vi "Pipeline Boolean Signal.vi"(7 "reset":bool, 10 "delay":fxp<+,5,5>, 11 "input signal":bool) -> (3 "output signal":bool)   [LabVIEW 2018]
doc: "Provide controlled delay for boolean signal."
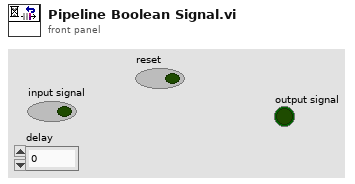
[diagram p1: front panel]
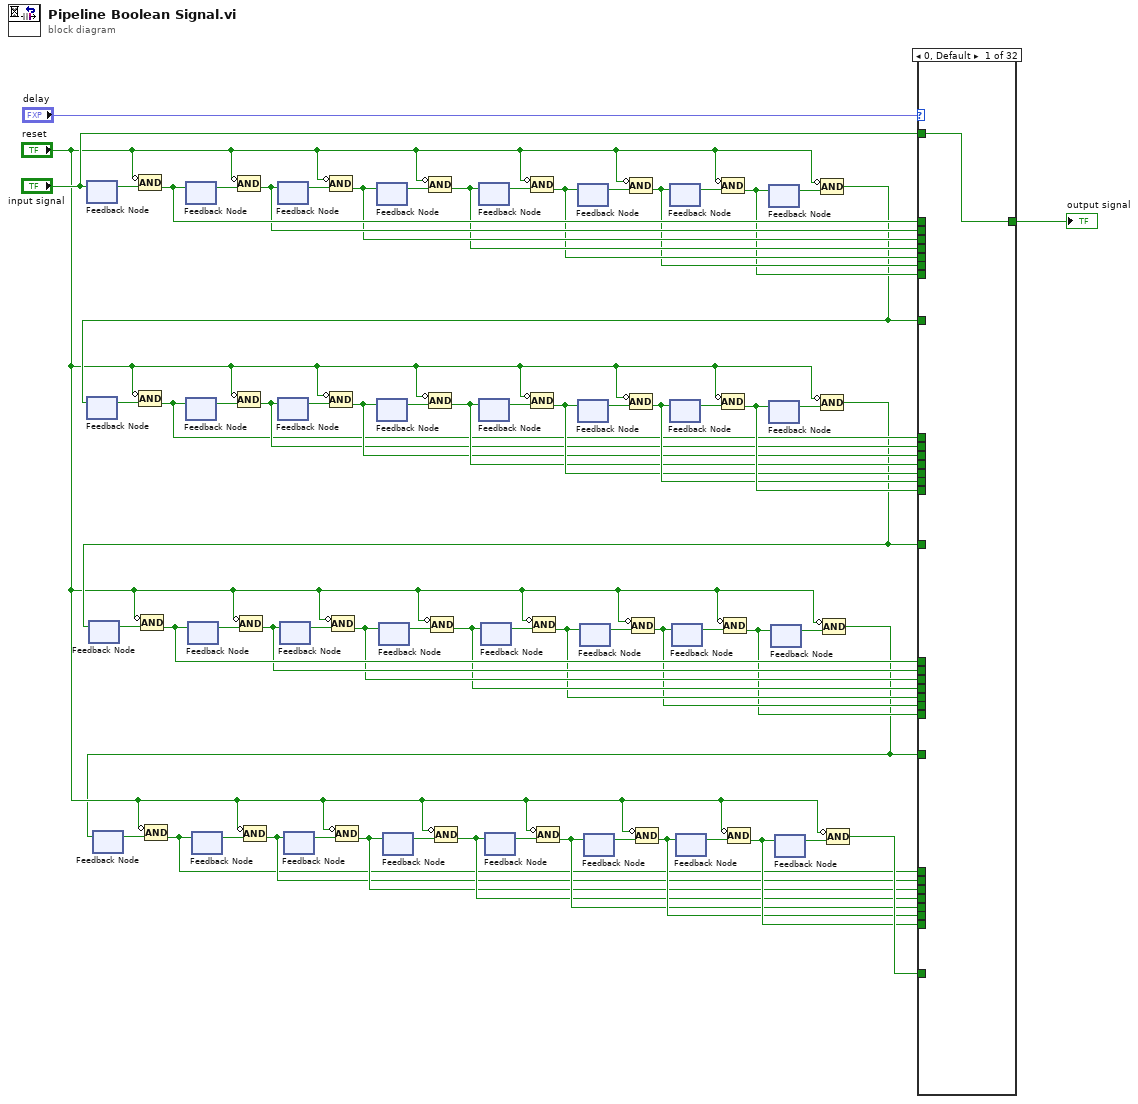
[diagram p0: block diagram]
diagram:
  n1 = feedback-in #1("input signal") -> ()
  n2 = feedback #1() -> (w65:bool)  [unwired: 1 in]
  n3 = feedback #2() -> (w41:bool)  [unwired: 1 in]
  n4 = feedback #3() -> (w31:bool)  [unwired: 1 in]
  n5 = feedback #4() -> (w6:bool)  [unwired: 1 in]
  n6 = Compound Arithmetic op=AND(invert "reset", w65) -> (w64:bool)
  n7 = Compound Arithmetic op=AND(invert "reset", w41) -> (w42:bool)
  n8 = Compound Arithmetic op=AND(invert "reset", w31) -> (w30:bool)
  n9 = Compound Arithmetic op=AND(invert "reset", w6) -> (w7:bool)
  n10 = feedback #5() -> (w68:bool)  [unwired: 1 in]
  n11 = feedback-in #5(w64) -> ()
  n12 = feedback #6() -> (w38:bool)  [unwired: 1 in]
  n13 = feedback-in #6(w42) -> ()
  n14 = feedback #7() -> (w34:bool)  [unwired: 1 in]
  n15 = feedback-in #7(w30) -> ()
  n16 = feedback #8() -> (w3:bool)  [unwired: 1 in]
  n17 = feedback-in #8(w7) -> ()
  n18 = Compound Arithmetic op=AND(invert "reset", w68) -> (w63:bool)
  n19 = Compound Arithmetic op=AND(invert "reset", w38) -> (w43:bool)
  n20 = Compound Arithmetic op=AND(invert "reset", w34) -> (w29:bool)
  n21 = Compound Arithmetic op=AND(invert "reset", w3) -> (w8:bool)
  n22 = feedback #9() -> (w67:bool)  [unwired: 1 in]
  n23 = feedback-in #9(w63) -> ()
  n24 = feedback #10() -> (w39:bool)  [unwired: 1 in]
  n25 = feedback-in #10(w43) -> ()
  n26 = feedback #11() -> (w33:bool)  [unwired: 1 in]
  n27 = feedback-in #11(w29) -> ()
  n28 = feedback #12() -> (w4:bool)  [unwired: 1 in]
  n29 = feedback-in #12(w8) -> ()
  n30 = Compound Arithmetic op=AND(invert "reset", w67) -> (w62:bool)
  n31 = Compound Arithmetic op=AND(invert "reset", w39) -> (w44:bool)
  n32 = Compound Arithmetic op=AND(invert "reset", w33) -> (w28:bool)
  n33 = Compound Arithmetic op=AND(invert "reset", w4) -> (w9:bool)
  n34 = feedback #13() -> (w66:bool)  [unwired: 1 in]
  n35 = feedback-in #13(w62) -> ()
  n36 = feedback #14() -> (w40:bool)  [unwired: 1 in]
  n37 = feedback-in #14(w44) -> ()
  n38 = feedback #15() -> (w32:bool)  [unwired: 1 in]
  n39 = feedback-in #15(w28) -> ()
  n40 = feedback #16() -> (w5:bool)  [unwired: 1 in]
  n41 = feedback-in #16(w9) -> ()
  n42 = Compound Arithmetic op=AND(invert "reset", w66) -> (w57:bool)
  n43 = Compound Arithmetic op=AND(invert "reset", w40) -> (w49:bool)
  n44 = Compound Arithmetic op=AND(invert "reset", w32) -> (w23:bool)
  n45 = Compound Arithmetic op=AND(invert "reset", w5) -> (w14:bool)
  n46 = feedback #17() -> (w61:bool)  [unwired: 1 in]
  n47 = feedback-in #17(w57) -> ()
  n48 = feedback #18() -> (w45:bool)  [unwired: 1 in]
  n49 = feedback-in #18(w49) -> ()
  n50 = feedback #19() -> (w27:bool)  [unwired: 1 in]
  n51 = feedback-in #19(w23) -> ()
  n52 = feedback #20() -> (w10:bool)  [unwired: 1 in]
  n53 = feedback-in #20(w14) -> ()
  n54 = Compound Arithmetic op=AND(invert "reset", w61) -> (w56:bool)
  n55 = Compound Arithmetic op=AND(invert "reset", w45) -> (w50:bool)
  n56 = Compound Arithmetic op=AND(invert "reset", w27) -> (w22:bool)
  n57 = Compound Arithmetic op=AND(invert "reset", w10) -> (w15:bool)
  n58 = feedback #21() -> (w58:bool)  [unwired: 1 in]
  n59 = feedback-in #21(w56) -> ()
  n60 = feedback #22() -> (w48:bool)  [unwired: 1 in]
  n61 = feedback-in #22(w50) -> ()
  n62 = feedback #23() -> (w24:bool)  [unwired: 1 in]
  n63 = feedback-in #23(w22) -> ()
  n64 = feedback #24() -> (w13:bool)  [unwired: 1 in]
  n65 = feedback-in #24(w15) -> ()
  n66 = Compound Arithmetic op=AND(invert "reset", w58) -> (w55:bool)
  n67 = Compound Arithmetic op=AND(invert "reset", w48) -> (w51:bool)
  n68 = Compound Arithmetic op=AND(invert "reset", w24) -> (w21:bool)
  n69 = Compound Arithmetic op=AND(invert "reset", w13) -> (w16:bool)
  n70 = feedback #25() -> (w59:bool)  [unwired: 1 in]
  n71 = feedback-in #25(w55) -> ()
  n72 = feedback #26() -> (w47:bool)  [unwired: 1 in]
  n73 = feedback-in #26(w51) -> ()
  n74 = feedback #27() -> (w25:bool)  [unwired: 1 in]
  n75 = feedback-in #27(w21) -> ()
  n76 = feedback #28() -> (w12:bool)  [unwired: 1 in]
  n77 = feedback-in #28(w16) -> ()
  n78 = Compound Arithmetic op=AND(invert "reset", w59) -> (w54:bool)
  n79 = Compound Arithmetic op=AND(invert "reset", w47) -> (w52:bool)
  n80 = Compound Arithmetic op=AND(invert "reset", w25) -> (w20:bool)
  n81 = Compound Arithmetic op=AND(invert "reset", w12) -> (w17:bool)
  n82 = feedback #29() -> (w60:bool)  [unwired: 1 in]
  n83 = feedback-in #29(w54) -> ()
  n84 = feedback #30() -> (w46:bool)  [unwired: 1 in]
  n85 = feedback-in #30(w52) -> ()
  n86 = feedback #31() -> (w26:bool)  [unwired: 1 in]
  n87 = feedback-in #31(w20) -> ()
  n88 = feedback #32() -> (w11:bool)  [unwired: 1 in]
  n89 = feedback-in #32(w17) -> ()
  n90 = Compound Arithmetic op=AND(invert "reset", w60) -> (w37:bool)
  n91 = feedback-in #2(w37) -> ()
  n92 = Compound Arithmetic op=AND(invert "reset", w46) -> (w19:bool)
  n93 = feedback-in #3(w19) -> ()
  n94 = Compound Arithmetic op=AND(invert "reset", w26) -> (w1:bool)
  n95 = feedback-in #4(w1) -> ()
  n96 = Compound Arithmetic op=AND(invert "reset", w11) -> (w18:bool)
  n97 = case shown="0, Default" "delay" {
    tunnel: w64 -> [_ w70 _ _ _ _ _ _ _ _ _ _ _ _ _ _ _ _ _ _ _ _ _ _ _ _ _ _ _ _ _ _]
    tunnel: w63 -> [_ _ w71 _ _ _ _ _ _ _ _ _ _ _ _ _ _ _ _ _ _ _ _ _ _ _ _ _ _ _ _ _]
    tunnel: w62 -> [_ _ _ w72 _ _ _ _ _ _ _ _ _ _ _ _ _ _ _ _ _ _ _ _ _ _ _ _ _ _ _ _]
    tunnel: w57 -> [_ _ _ _ w73 _ _ _ _ _ _ _ _ _ _ _ _ _ _ _ _ _ _ _ _ _ _ _ _ _ _ _]
    tunnel: w56 -> [_ _ _ _ _ w74 _ _ _ _ _ _ _ _ _ _ _ _ _ _ _ _ _ _ _ _ _ _ _ _ _ _]
    tunnel: w55 -> [_ _ _ _ _ _ w75 _ _ _ _ _ _ _ _ _ _ _ _ _ _ _ _ _ _ _ _ _ _ _ _ _]
    tunnel: w54 -> [_ _ _ _ _ _ _ w76 _ _ _ _ _ _ _ _ _ _ _ _ _ _ _ _ _ _ _ _ _ _ _ _]
    tunnel: [w69 w70 w71 w72 w73 w74 w75 w76 w77 w78 w79 w80 w81 w82 w83 w84 w85 w86 w87 w88 w89 w90 w91 w92 w93 w94 w95 w96 w97 w98 w99 w100] -> w53
    tunnel: w37 -> [_ _ _ _ _ _ _ _ w77 _ _ _ _ _ _ _ _ _ _ _ _ _ _ _ _ _ _ _ _ _ _ _]
    tunnel: w42 -> [_ _ _ _ _ _ _ _ _ w78 _ _ _ _ _ _ _ _ _ _ _ _ _ _ _ _ _ _ _ _ _ _]
    tunnel: w43 -> [_ _ _ _ _ _ _ _ _ _ w79 _ _ _ _ _ _ _ _ _ _ _ _ _ _ _ _ _ _ _ _ _]
    tunnel: w44 -> [_ _ _ _ _ _ _ _ _ _ _ w80 _ _ _ _ _ _ _ _ _ _ _ _ _ _ _ _ _ _ _ _]
    tunnel: w49 -> [_ _ _ _ _ _ _ _ _ _ _ _ w81 _ _ _ _ _ _ _ _ _ _ _ _ _ _ _ _ _ _ _]
    tunnel: w50 -> [_ _ _ _ _ _ _ _ _ _ _ _ _ w82 _ _ _ _ _ _ _ _ _ _ _ _ _ _ _ _ _ _]
    tunnel: w51 -> [_ _ _ _ _ _ _ _ _ _ _ _ _ _ w83 _ _ _ _ _ _ _ _ _ _ _ _ _ _ _ _ _]
    tunnel: w52 -> [_ _ _ _ _ _ _ _ _ _ _ _ _ _ _ w84 _ _ _ _ _ _ _ _ _ _ _ _ _ _ _ _]
    tunnel: "input signal" -> [w69 _ _ _ _ _ _ _ _ _ _ _ _ _ _ _ _ _ _ _ _ _ _ _ _ _ _ _ _ _ _ _]
    tunnel: w19 -> [_ _ _ _ _ _ _ _ _ _ _ _ _ _ _ _ w85 _ _ _ _ _ _ _ _ _ _ _ _ _ _ _]
    tunnel: w30 -> [_ _ _ _ _ _ _ _ _ _ _ _ _ _ _ _ _ w86 _ _ _ _ _ _ _ _ _ _ _ _ _ _]
    tunnel: w29 -> [_ _ _ _ _ _ _ _ _ _ _ _ _ _ _ _ _ _ w87 _ _ _ _ _ _ _ _ _ _ _ _ _]
    tunnel: w28 -> [_ _ _ _ _ _ _ _ _ _ _ _ _ _ _ _ _ _ _ w88 _ _ _ _ _ _ _ _ _ _ _ _]
    tunnel: w23 -> [_ _ _ _ _ _ _ _ _ _ _ _ _ _ _ _ _ _ _ _ w89 _ _ _ _ _ _ _ _ _ _ _]
    tunnel: w22 -> [_ _ _ _ _ _ _ _ _ _ _ _ _ _ _ _ _ _ _ _ _ w90 _ _ _ _ _ _ _ _ _ _]
    tunnel: w21 -> [_ _ _ _ _ _ _ _ _ _ _ _ _ _ _ _ _ _ _ _ _ _ w91 _ _ _ _ _ _ _ _ _]
    tunnel: w20 -> [_ _ _ _ _ _ _ _ _ _ _ _ _ _ _ _ _ _ _ _ _ _ _ w92 _ _ _ _ _ _ _ _]
    tunnel: w1 -> [_ _ _ _ _ _ _ _ _ _ _ _ _ _ _ _ _ _ _ _ _ _ _ _ w93 _ _ _ _ _ _ _]
    tunnel: w7 -> [_ _ _ _ _ _ _ _ _ _ _ _ _ _ _ _ _ _ _ _ _ _ _ _ _ w94 _ _ _ _ _ _]
    tunnel: w8 -> [_ _ _ _ _ _ _ _ _ _ _ _ _ _ _ _ _ _ _ _ _ _ _ _ _ _ w95 _ _ _ _ _]
    tunnel: w9 -> [_ _ _ _ _ _ _ _ _ _ _ _ _ _ _ _ _ _ _ _ _ _ _ _ _ _ _ w96 _ _ _ _]
    tunnel: w14 -> [_ _ _ _ _ _ _ _ _ _ _ _ _ _ _ _ _ _ _ _ _ _ _ _ _ _ _ _ w97 _ _ _]
    tunnel: w15 -> [_ _ _ _ _ _ _ _ _ _ _ _ _ _ _ _ _ _ _ _ _ _ _ _ _ _ _ _ _ w98 _ _]
    tunnel: w16 -> [_ _ _ _ _ _ _ _ _ _ _ _ _ _ _ _ _ _ _ _ _ _ _ _ _ _ _ _ _ _ w99 _]
    tunnel: w17 -> [_ _ _ _ _ _ _ _ _ _ _ _ _ _ _ _ _ _ _ _ _ _ _ _ _ _ _ _ _ _ _ w100]
    tunnel: w18 -> [_ _ _ _ _ _ _ _ _ _ _ _ _ _ _ _ _ _ _ _ _ _ _ _ _ _ _ _ _ _ _ _]
    frame 0, Default {
    }
    frame 1 {
    }
    frame 2 {
    }
    frame 3 {
    }
    frame 4 {
    }
    frame 5 {
    }
    frame 6 {
    }
    frame 7 {
    }
    frame 8 {
    }
    frame 9 {
    }
    frame 10 {
    }
    frame 11 {
    }
    frame 12 {
    }
    frame 13 {
    }
    frame 14 {
    }
    frame 15 {
    }
    frame 16 {
    }
    frame 17 {
    }
    frame 18 {
    }
    frame 19 {
    }
    frame 20 {
    }
    frame 21 {
    }
    frame 22 {
    }
    frame 23 {
    }
    frame 24 {
    }
    frame 25 {
    }
    frame 26 {
    }
    frame 27 {
    }
    frame 28 {
    }
    frame 29 {
    }
    frame 30 {
    }
    frame 31 {
    }
  }
  "output signal" <- w53
